vi "wave_random_number.vi"() -> ()   [LabVIEW 2020]
panel:
  in  "phase":dbl
  in  "omega":dbl
  in  "stop2":bool
  out "Sinewave":dbl(graph)
  in  "stop":bool
  out "Waveform Chart":dbl(graph)
  # "Wave random number test"
  # "Sinewave random number"
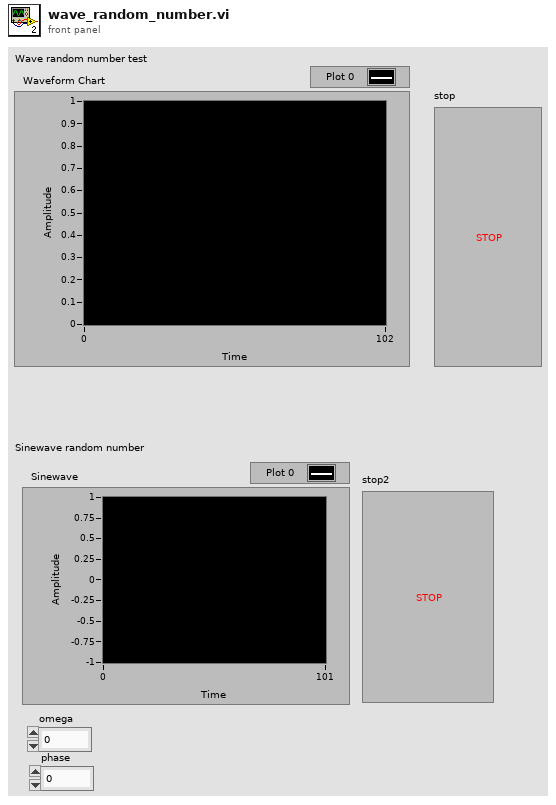
[diagram p1: front panel]
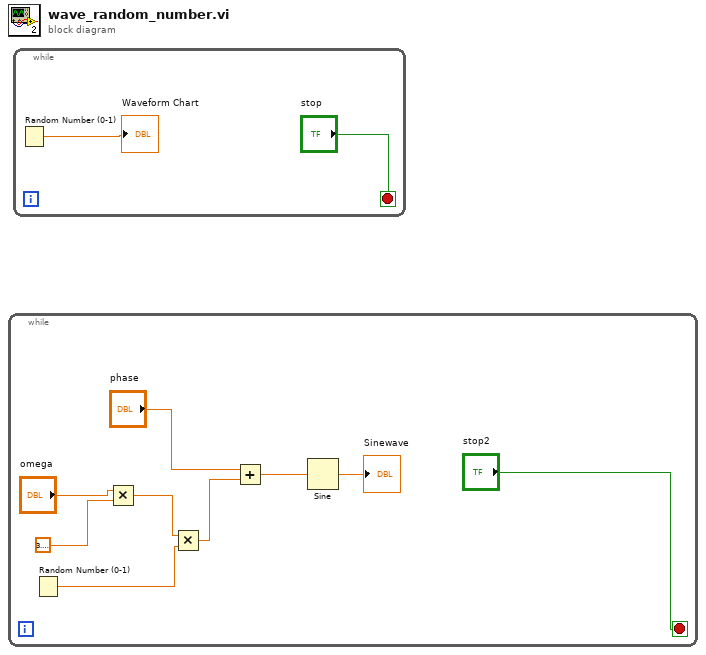
[diagram p0: block diagram]
diagram:
  n1 = while {
    stop <- "stop2" stop-if-true
    n2 = Random Number (0-1)() -> (number: 0 to 1=w1:dbl)
    n3 = Multiply(x="omega", y=3.141592653589793) -> (x*y=w2:dbl)
    n4 = Multiply(x=w2, y=w1) -> (x*y=w8:dbl)
    n5 = Add(x="phase", y=w8) -> (x+y=w7:dbl)
    n6 = Sine(x=w7) -> (sin(x)=→"Sinewave":dbl)
  }
  n7 = while {
    stop <- "stop" stop-if-true
    n8 = Random Number (0-1)() -> (number: 0 to 1=→"Waveform Chart":dbl)
  }
